vi "UpdateTimestamp.vi"(7 "Age Limit [s]":dbl, 8 "Error In":errorcluster, 10 "Timestamp":timestamp, 11 "Indicator Refnum":refnum<vi>) -> (0 "Error Out":errorcluster)   [LabVIEW 2017, in "Client.lvlib" / "UI_API.lvlib"]
uses:
  UI_API.lvlib
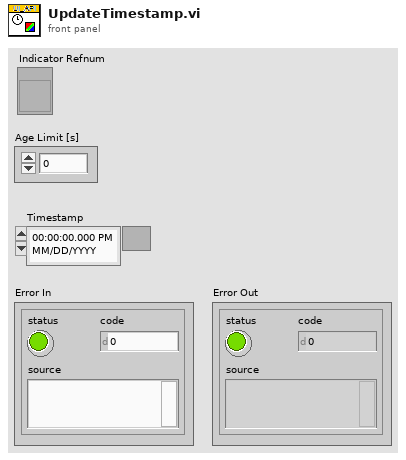
[diagram p1: front panel]
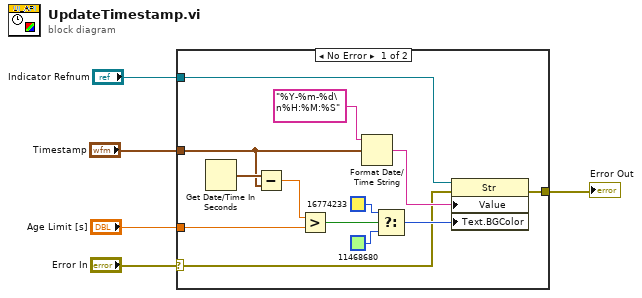
[diagram p0: block diagram]
diagram:
  n1 = case shown="No Error" "Error In" {
    selector: "Error In" -> [w7 w19]
    tunnel: "Indicator Refnum" -> [w17 _]
    tunnel: "Timestamp" -> [w14 _]
    tunnel: "Age Limit [s]" -> [w12 _]
    tunnel: [w6 w19] -> w1
    frame No Error {
      n2 = Get Date/Time In Seconds() -> (seconds since 1Jan1904=w15:timestamp)
      n3 = Subtract(x=w15, y=w14) -> (x-y=w13:dbl)
      n4 = Greater?(x=w13, y=w12) -> (0:w9:bool)
      n5 = Format Date/Time String(time format string (%c)="%Y-%m-%d\n%H:%M:%S", seconds (now)=w14) -> (date/time string=w18:string)  [unwired: 1 in]
      n6 = Select(t=u32 16774233, s=w9, f=u32 11468680) -> (s? t:f=w8:u32)
      n7 = property class="Str"(reference=w17, error in=w7, "Value"=w18, "Text.BGColor"=w8) -> (error out=w6:errorcluster)  [unwired: 1 out]
    }
    frame Error {
    }
  }
  "Error Out" <- w1
